vi "Test1.vi"() -> ()   [LabVIEW 2017, in "ModBUS.lvlib" / "Modbus.lvclass"]
uses:
  Modbus.lvclass
  ASCII/ASCII.lvclass
panel:
  out "x = y? 2":bool[](array[boolean])
  out "Data":i16[](array[numeric]) format="%.0x"
  out "x = y?":bool
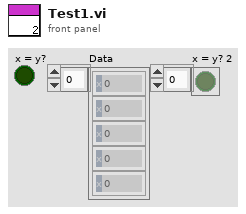
[diagram p1: front panel]
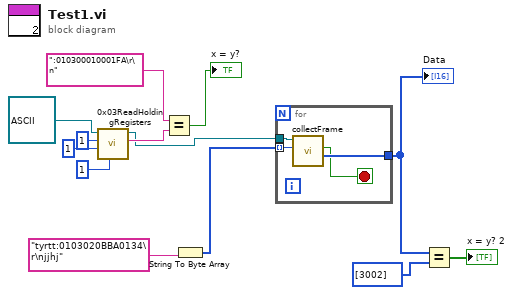
[diagram p0: block diagram]
diagram:
  n1 = call-dynamic "0x03ReadHoldingRegisters.vi"("Length 2"=u16 1, "Register"=u16 1, "Addressc"=u8 1, "ASCII in"=refnum<class "ASCII.lvclass"> refnum ("ASCII.lvclass")) -> ("Frame"=w9:string, "ASCII out"=w4:refnum<class "ASCII.lvclass">)  [unwired: 5 in, 1 out]
  n2 = Equal?(x=":010300010001FA\r\n" ("Frame 2"), y=w9) -> (x = y?=→"x = y?":bool)
  n3 = String To Byte Array(string="tyrtt:0103020BBA0134\r\njjhj" ("Frame 2")) -> (unsigned byte array=w5:u8[])
  n4 = for {
    tunnel: w5 -> [w17] mode=indexing
    tunnel: w4 -> [w16]
    tunnel: [w15] -> w2
    stop <- w14 stop-if-true
    n5 = call-dynamic "collectFrame.vi"("byte"=w17, "ASCII in"=w16) -> ("Data"=w15:i16[], "Finished"=w14:bool)  [unwired: 5 in, 3 out]
  }
  "Data" <- w2
  n6 = Equal?(x=w2, y=i16[] [3002] ("Data")) -> (x = y?=→"x = y? 2":bool[])
